vi "Local Loop.vi"() -> ()   [LabVIEW 2012]
uses:
  <vilib>/Platform/TimedLoop/XDataNode/timing_clust.ctl
  <vilib>/Platform/TimedLoop/XDataNode/nitl_modes.ctl
  <vilib>/Platform/TimedLoop/XDataNode/wakeup.ctl
  <vilib>/Platform/TimedLoop/XDataNode/XDataNode.xnode
  <vilib>/Platform/TimedLoop/XDataNode/XDNodeRunTimeDep.lvlib
panel:
  out "VTan_Cmd":dbl(slide) scale=-10.0..10.0
  out "VAng_Cmd":dbl(slide) scale=-10.0..10.0
  in  "PID gains":cluster{"P":dbl, "I":dbl, "D":dbl}
  in  "stop?":bool
  out "Error Out":errorcluster
  in  "Error In":errorcluster
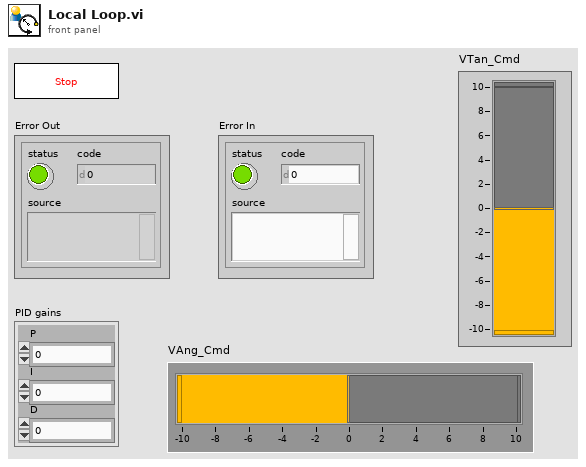
[diagram p1: front panel]
types:
  T1 = typedef "XDNodeRunTimeDep.lvlib/timing_clust.ctl" = cluster{"Expected End [f-1]":u64, "Actual End [f-1]":u64, "Finished Late? [f-1]":bool, "Expected End [i-1]":u64, "Actual End [i-1]":u64, "Finished Late? [i-1]":bool, "Expected Start [i]":u64, "Actual Start [i]":u64, "Expected Start [f]":u64, "Actual Start [f]":u64, "Source Name":string, "Structure Name":string, "Period":i64, "Deadline":i64, "Offset":i64, "Start":i64, "Priority":i32, "Timeout":i32, "Mode":T2, "Wakeup Reason":T3, "Error":errorcluster, "Source Type":string, "Secondary Source Type":string, "Global End Time":u64, "Global Start Time":u64, "Frame Duration":u64, "Iteration Duration":u64, "Assigned CPU":i32, "I/O Scan Engine Mode":u32}
  T2 = typedef "XDNodeRunTimeDep.lvlib/nitl_modes.ctl" = enum32{"No Change", "Process missed periods, maintain original phase", "Discard missed periods, maintain original phase", "Process missed periods, ignore original phase", "Discard missed periods, ignore original phase"}
  T3 = typedef "XDNodeRunTimeDep.lvlib/wakeup.ctl" = enum32{"Normal", "Aborted", "Asynchronous wakeup", "Timing source error", "Timed loop error", "Timeout"}
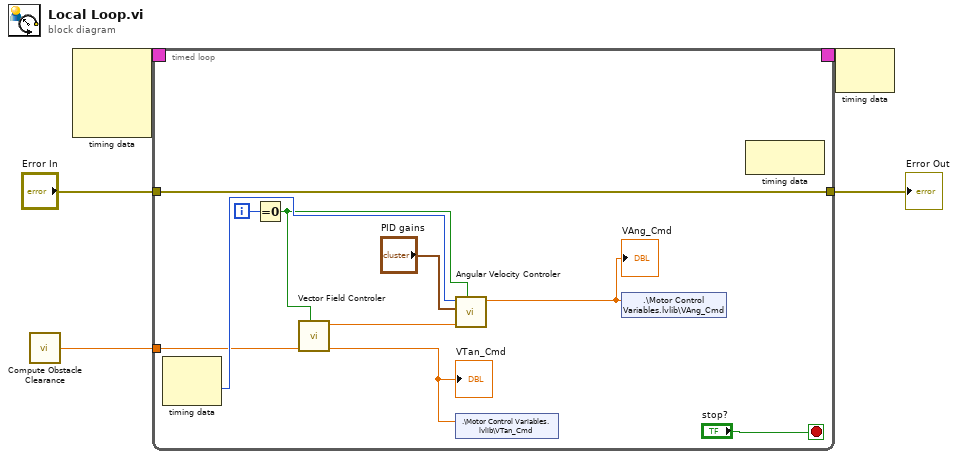
[diagram p0: block diagram]
diagram:
  n1 = call "Compute Obstacle Clearance.vi"() -> ("obstacle clearance (m)"=w1:dbl)  [unwired: 1 in]
  n2 = node-c288() -> (w5:T1)  [unwired: 4 in]
  n3 = timed-loop {
    timing: w5 -> [_]
    timing-out: [_] -> w4
    tunnel: "Error In" -> [w14]
    tunnel: [w14] -> w2
    tunnel: w1 -> [w9]
    i -> [w13]
    stop <- "stop?" stop-if-true
    n4 = node-c288() -> (w11:i64)  [unwired: 1 in, 1 out]
    n5 = Equal To 0?(x=w13) -> (x = 0?=w8:bool)
    n6 = call "Vector Field Controler.vi"("Initialize?"=w8, "obstacle clearance (m)"=w9) -> ("VTan_Cmd"=w7:dbl, "Command Heading"=w6:dbl)  [unwired: 8 in]
    "VTan_Cmd" <- w7
    n7 = call "Angular Velocity Controler.vi"("reinitialize? (F)"=w8, "Command Heading"=w6, "PID gains"="PID gains", "Period"=w11) -> ("VAng_Cmd"=w10:dbl)  [unwired: 7 in]
    "VAng_Cmd" <- w10
    n8 = shared-variable ".\\Motor Control Variables.lvlib\\VTan_Cmd"(w7) -> ()  [unwired: 1 in, 1 out]
    n9 = shared-variable ".\\Motor Control Variables.lvlib\\VAng_Cmd"(w10) -> ()  [unwired: 1 in, 1 out]
    n10 = node-c288() -> ()  [unwired: 1 in, 1 out]
  }
  "Error Out" <- w2
  n11 = node-c288(w4) -> ()  [unwired: 1 out]
